vi "Handle Graph Settings.vi"(6 "Table Setting Name in":string, 7 "Write Ctl? (F:Read)":bool, 8 "error in (no error)":errorcluster, 9 "Table Ref":refnum<vi>, 11 "Save Restore Settings in":refnum<class "Save Restore Settings.lvclass">) -> (0 "error out":errorcluster, 1 "Sub Controls":T1[](array[typedef]), 3 "Save Restore Settings out":refnum<class "Save Restore Settings.lvclass">)   [LabVIEW 2016, in "Save Restore Settings.lvclass"]
uses:
  <userlib>/_MGI/Application Control/MGI Save Restore Settings/Save Restore Settings.lvclass
  <userlib>/_MGI/Application Control/MGI Save Restore Settings/Control Info.ctl
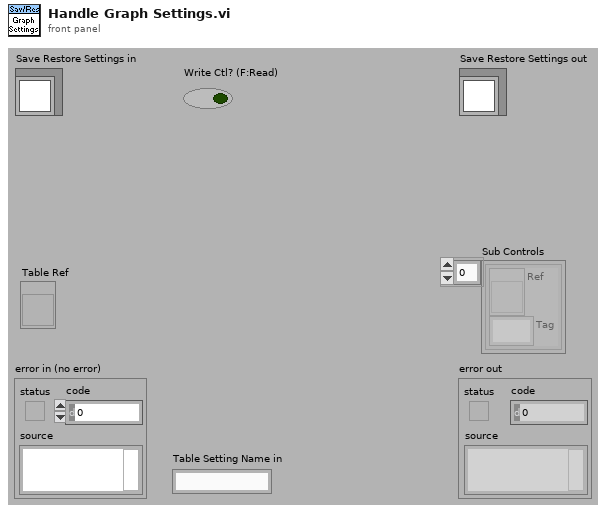
[diagram p1: front panel]
types:
  T1 = typedef "Save Restore Settings.lvclass/Control Info.ctl" = cluster{"Ref":refnum<vi>, "Tag":string}
  T2 = cluster{"XScaleIdx":u32, "YScaleIdx":u32, "Info":cluster{"Plot Color":u32, "Plot Interpolation":u8, "Point Style":u8, "Line Style":u8, "Fill/Pt. Color":u32, "Line Width":u8, "Bar Plot Style":u8, "Fill To":i16}}
  T3 = cluster{"Plot Color":u32, "Plot Interpolation":u8, "Point Style":u8, "Line Style":u8, "Fill/Pt. Color":u32, "Line Width":u8, "Bar Plot Style":u8, "Fill To":i16}
  T4 = cluster{"XScaleIdx":u32, "YScaleIdx":u32, "Info":cluster{"Plot Color":u32, "Plot Interpolation":u8, "Point Style":u8, "Line Style":u8, "Fill/Pt. Color":u32, "Line Width":u8, "Bar Plot Style":u8, "Fill To":i16}}[]
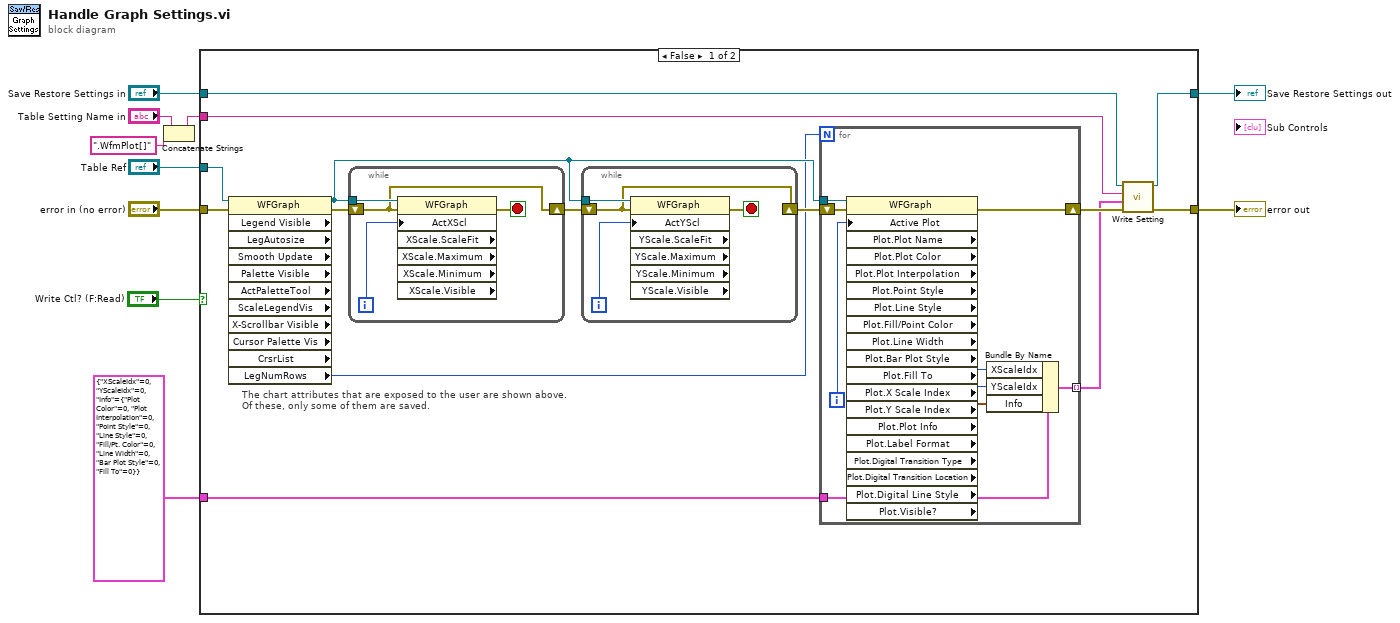
[diagram p0: block diagram]
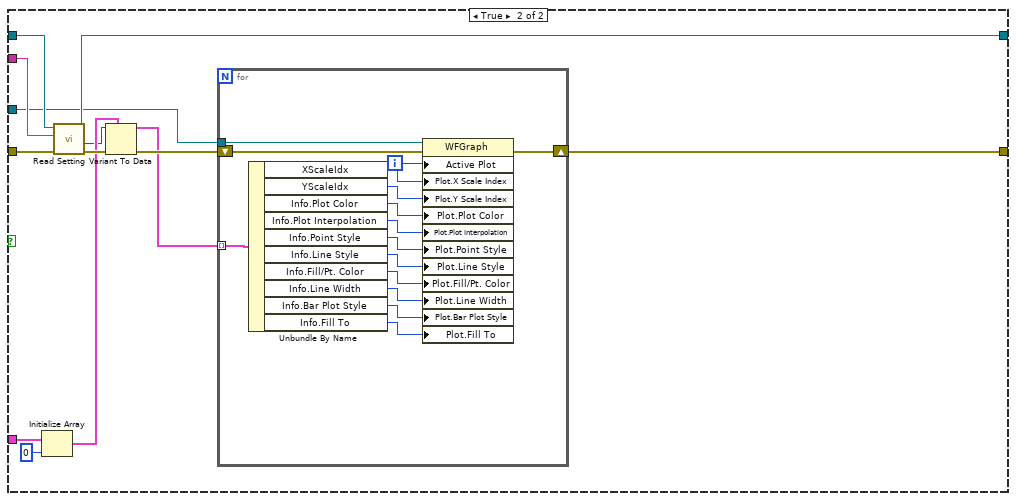
[diagram p2: hidden frame]
diagram:
  n1 = Concatenate Strings("Table Setting Name in", ".WfmPlot[]" ("string")) -> (w2:string)
  n2 = case shown="False" "Write Ctl? (F:Read)" {
    tunnel: "Table Ref" -> [w24 w45]
    tunnel: "error in (no error)" -> [w23 w53]
    tunnel: "Save Restore Settings in" -> [w22 w51]
    tunnel: [w21 w50] -> w7
    tunnel: [w20 w43] -> w6
    tunnel: w2 -> [w12 w52]
    tunnel: T2 {"XScaleIdx"=0, "YScaleIdx"=0, "Info"={"Plot Color"=0, "Plot Interpolation"=0, "Point Style"=0, "Line Style"=0, "Fill/Pt. Color"=0, "Line Width"=0, "Bar Plot Style"=0, "Fill To"=0}} ("output cluster") -> [w11 w49]
    frame False {
      # "The chart attributes that are exposed to the user are shown above.\nOf these, only some of them are saved."
      n3 = property class="WFGraph" props=["Legend Visible", "LegAutosize", "Smooth Update", "Palette Visible", "ActPaletteTool", "ScaleLegendVis", "X-Scrollbar Visible", "Cursor Palette Vis", "CrsrList", "LegNumRows"](reference=w24, error in=w23) -> (reference out=w15:refnum<vi>, error out=w19:errorcluster, "LegNumRows"=w13:u32)  [unwired: 9 out]
      n4 = while {
        tunnel: w15 -> [w40]
        shift-right: [w39] -> w18
        shift-left: w19 -> [w39]
        i -> [w38]
        stop <- w41 stop-if-true
        n5 = property class="WFGraph" props=["ActXScl", "XScale", "ScaleFit", "XScale", "Maximum", "XScale", "Minimum", "XScale", "Visible"](reference=w40, error in=w39, "ActXScl"=w38) -> (error out=w41:errorcluster)  [unwired: 5 out]
      }
      n6 = while {
        tunnel: w15 -> [w36]
        shift-right: [w35] -> w17
        shift-left: w18 -> [w35]
        i -> [w34]
        stop <- w37 stop-if-true
        n7 = property class="WFGraph" props=["ActYScl", "YScale", "ScaleFit", "YScale", "Maximum", "YScale", "Minimum", "YScale", "Visible"](reference=w36, error in=w35, "ActYScl"=w34) -> (error out=w37:errorcluster)  [unwired: 5 out]
      }
      n8 = for {
        N: w13 -> [_]
        shift-right: [w28] -> w16
        shift-left: w17 -> [w29]
        tunnel: w15 -> [w31]
        tunnel: w11 -> [w33]
        tunnel: [w32] -> w14 mode=indexing
        i -> [w30]
        n9 = property class="WFGraph" props=["Active Plot", "Plot", "Plot Name", "Plot", "Plot Color", "Plot", "Plot Interpolation", "Plot", "Point Style", "Plot", "Line Style", "Plot", "Fill/Point Color", "Plot", "Line Width", "Plot", "Bar Plot Style", "Plot", "Fill To", "Plot", "X Scale Index", "Plot", "Y Scale Index", "Plot", "Plot Info", "Plot", "Label Format", "Plot", "Digital Transition Type", "Plot", "Digital Transition Location", "Plot", "Digital Line Style", "Plot", "Visible?"](reference=w31, error in=w29, "Active Plot"=w30) -> (error out=w28:errorcluster, "Plot.X Scale Index"=w26:u32, "Plot.Y Scale Index"=w25:u32, "Plot.Plot Info"=w27:T3)  [unwired: 15 out]
        n10 = Bundle By Name(cluster=w33, "XScaleIdx"=w26, "YScaleIdx"=w25, "Info"=w27) -> (w32:T2)
      }
      n11 = call-dynamic "Write Setting.vi"("error in (no error)"=w16, "Tag Attribute"=w14, "Tag Name"=w12, "Save Restore Settings in"=w22) -> ("error out"=w20:errorcluster, "Save Restore Settings out"=w21:refnum<class "Save Restore Settings.lvclass">)  [unwired: 6 in]
    }
    frame True {
      n12 = Initialize Array(w49, 0 ("dimension size")) -> (w47:T4)
      n13 = call-dynamic "Read Setting.vi"("error in (no error)"=w53, "Tag Name"=w52, "Save Restore Settings in"=w51) -> ("error out"=w54:errorcluster, "Tag Attribute"=w46:variant, "Save Restore Settings out"=w50:refnum<class "Save Restore Settings.lvclass">)  [unwired: 6 in]
      n14 = Variant To Data(error in=w54, type=w47, Variant=w46) -> (data=w42:T4, error out=w44:errorcluster)
      n15 = for {
        shift-right: [w67] -> w43
        shift-left: w44 -> [w68]
        tunnel: w45 -> [w69]
        tunnel: w42 -> [w65] mode=indexing
        i -> [w66]
        n16 = Unbundle By Name(w65) -> ("XScaleIdx"=w64:u32, "YScaleIdx"=w63:u32, "Info.Plot Color"=w62:u32, "Info.Plot Interpolation"=w61:u8, "Info.Point Style"=w60:u8, "Info.Line Style"=w59:u8, "Info.Fill/Pt. Color"=w58:u32, "Info.Line Width"=w57:u8, "Info.Bar Plot Style"=w56:u8, "Info.Fill To"=w55:i16)
        n17 = property class="WFGraph"(reference=w69, error in=w68, "Active Plot"=w66, "Plot.X Scale Index"=w64, "Plot.Y Scale Index"=w63, "Plot.Plot Color"=w62, "Plot.Plot Interpolation"=w61, "Plot.Point Style"=w60, "Plot.Line Style"=w59, "Plot.Fill/Pt. Color"=w58, "Plot.Line Width"=w57, "Plot.Bar Plot Style"=w56, "Plot.Fill To"=w55) -> (error out=w67:errorcluster)  [unwired: 1 out]
      }
    }
  }
  "error out" <- w6
  "Save Restore Settings out" <- w7
